vi "checkgyro.vi"(8 "error in (no error)":errorcluster) -> ()   [LabVIEW 2013]
panel:
  out "Data Out":string
  out "Array":T1(array[cluster])
  in  "Steps":i32
  in  "milliseconds/cycle":u32
  out "Gauge":cluster{dbl, dbl}(knob)={0.0, 185.10371008048537} scale=0.0..360.0
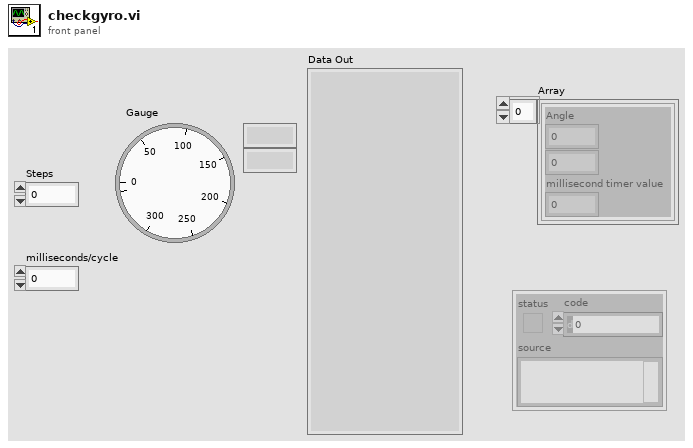
[diagram p1: front panel]
types:
  T1 = cluster{"Angle":dbl, i32, "millisecond timer value":u32}[]
  T2 = typedef "WPI_GyroDevRef.ctl" = cluster{"DevStatus":errorcluster, "Analog Module":T3, "Analog Channel":T4, "Offset":dbl, "Gain (VoltsPerDegree/Second)":dbl}
  T3 = typedef "FPGA_TypedefAnalogModule.ctl" = enum16{"Analog Module 1", "Analog Module 2"}
  T4 = typedef "FPGA_AIChannel.ctl" = enum8{"AI 1", "AI 2", "AI 3", "AI 4", "AI 5", "AI 6", "AI 7", "AI 8", "Invalid"}
  T5 = typedef "WPI_ServoDeviceRef.ctl" = cluster{"DeviceStatus":errorcluster, "Digital Module":T6, "PWM Channel":T7, "DeadBand":T8}
  T6 = typedef "FPGA_TypedefDigitalModule.ctl" = enum16{"Digital Module 1", "Digital Module 2"}
  T7 = typedef "FPGA_DIOPWMChannel.ctl" = enum8{"PWM 1", "PWM 2", "PWM 3", "PWM 4", "PWM 5", "PWM 6", "PWM 7", "PWM 8", "PWM 9", "PWM 10", "Invalid"}
  T8 = typedef "WPI_PWMDeadband.ctl" = cluster{"Name":string, "maxPositivePwm":i32, "minPositivePwm":i32, "centerPwm":i32, "maxNegativePwm":i32, "minNegativePwm":i32, "angularRange":u16}
  T9 = cluster{"Angle":dbl, i32, "millisecond timer value":u32}
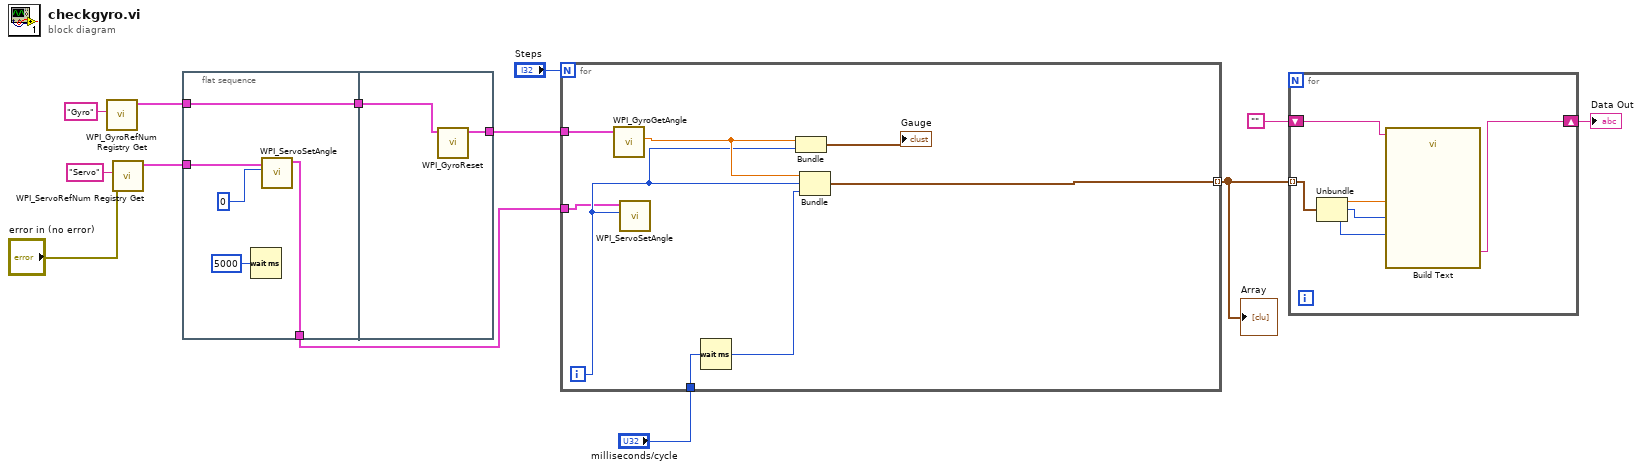
[diagram p0: block diagram]
diagram:
  n1 = call <vilib>:"WPI_GyroRefNum Registry Get.vi"("refnum name"="Gyro") -> ("GyroDevRef"=w12:T2)  [unwired: 9 in, 1 out]
  n2 = call <vilib>:"WPI_ServoRefNum Registry Get.vi"("error in (no error)"="error in (no error)", "refnum name"="Servo") -> ("ServoDeviceRef"=w13:T5)  [unwired: 8 in, 1 out]
  n3 = flat-sequence {
    tunnel: w13 -> [w18]
    tunnel: w12 -> [w16]
    tunnel: [w16] -> w11
    tunnel: [w15] -> w9
    tunnel: w11 -> [w20]
    tunnel: [w19] -> w10
    frame #0 {
      n4 = Wait (ms)(milliseconds to wait=u32 5000) -> ()  [unwired: 1 out]
      n5 = call <vilib>:"WPI_ServoSetAngle.vi"("Angle"=0, "ServoDeviceRef"=w18) -> ("ServoDeviceRef"=w15:T5)  [unwired: 8 in, 1 out]
    }
    frame #1 {
      n6 = call <vilib>:"WPI_GyroReset.vi"("GyroDevRef"=w20) -> ("GyroDevRef"=w19:T2)  [unwired: 9 in, 1 out]
    }
  }
  n7 = for {
    N: "Steps" -> [_]
    tunnel: w10 -> [w28]
    tunnel: w9 -> [w21]
    tunnel: "milliseconds/cycle" -> [w27]
    tunnel: [w25] -> w5 mode=indexing
    i -> [w23]
    n8 = call <vilib>:"WPI_GyroGetAngle.vi"("GyroDevRef"=w28) -> ("Angle"=w24:dbl)  [unwired: 7 in, 3 out]
    n9 = call <vilib>:"WPI_ServoSetAngle.vi"("Angle"=w23, "ServoDeviceRef"=w21) -> ()  [unwired: 8 in, 2 out]
    n10 = Wait (ms)(milliseconds to wait=w27) -> (millisecond timer value=w26:u32)
    n11 = Bundle("Angle"=w24, w23) -> (→"Gauge":cluster{"Angle":dbl, i32})  [unwired: 1 in]
    n12 = Bundle("Angle"=w24, w23, "millisecond timer value"=w26) -> (w25:T9)  [unwired: 1 in]
  }
  "Array" <- w5
  n13 = for {
    tunnel: w5 -> [w32] mode=indexing
    shift-right: [w33] -> w4
    shift-left: "" -> [w34]
    n14 = Unbundle(w32) -> ("Angle"=w31:dbl, w30:i32, "millisecond timer value"=w29:u32)
    n15 = call "Build Text"("Beginning Text"=w34, "gyro"=w31, "servo"=w30, "time"=w29) -> ("Result"=w33:string)  [unwired: 10 in, 1 out]
  }
  "Data Out" <- w4
